vi "Untitled 1.vi"() -> ()   [LabVIEW 2019]
uses:
  Generated_client/RPC Messages/helloworld_HelloRequest.ctl
  Generated_client/RPC Messages/helloworld_Person.ctl
  Generated_client/RPC Messages/helloworld_HelloReply.ctl
  Generated_client/Generated_client.lvlib
panel:
  out "error out":errorcluster
  out "Response Data":T1
  in  "Request Data":T2
  in  "address":string
  in  "error in":errorcluster
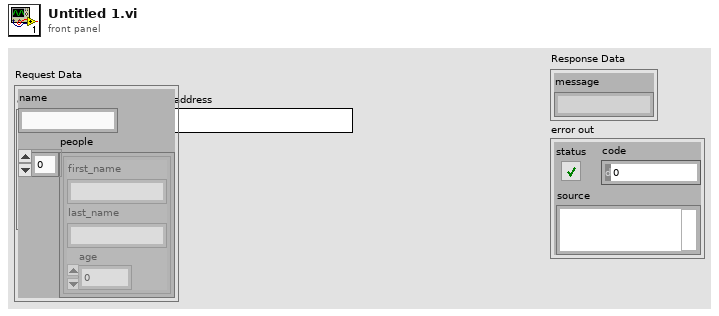
[diagram p1: front panel]
types:
  T1 = typedef "Generated_client.lvlib/helloworld_HelloReply.ctl" = cluster{"message":string}
  T2 = typedef "Generated_client.lvlib/helloworld_HelloRequest.ctl" = cluster{"name":string, "people":T3[]}
  T3 = typedef "Generated_client.lvlib/helloworld_Person.ctl" = cluster{"first_name":string, "last_name":string, "age":i32}
  T4 = typedef "grpc-lvsupport-release.lvlib/grpcId.ctl" = u64
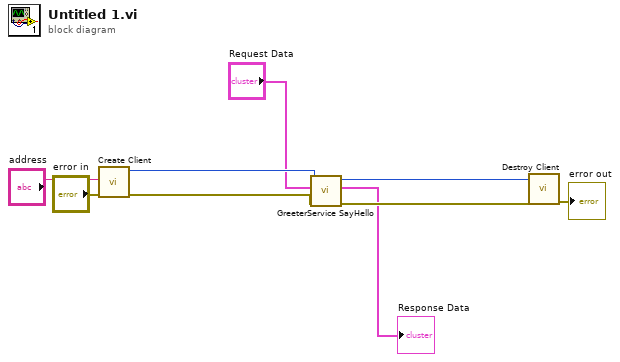
[diagram p0: block diagram]
diagram:
  n1 = call "Create Client.vi"("error in"="error in", "address"="address") -> ("error out"=w7:errorcluster, "gRPC ID Out"=w9:T4)  [unwired: 8 in]
  n2 = call "GreeterService SayHello.vi"("error in"=w7, "Request Data"="Request Data", "gRPC ID"=w9) -> ("error out"=w6:errorcluster, "Response Data"=→"Response Data":T1, "gRPC ID out"=w8:T4)  [unwired: 6 in]
  n3 = call "Destroy Client.vi"("error in"=w6, "gRPC ID"=w8) -> ("error out"=→"error out":errorcluster)  [unwired: 9 in]
